vi "PC_SetCommandTo_PLC.vi"(0 "VISA resource name":refnum<visa-resource-name>, 1 "Mode":enum16{"RTU", "ASCII"}(ring), 2 "PLC Address":u8, 3 "Resistor":i32, 4 "Selection":T1(ring), 5 "error in (no error)":errorcluster) -> (6 "VISA resource name out":refnum<visa-resource-name>, 8 "error out":errorcluster)   [LabVIEW 2015]
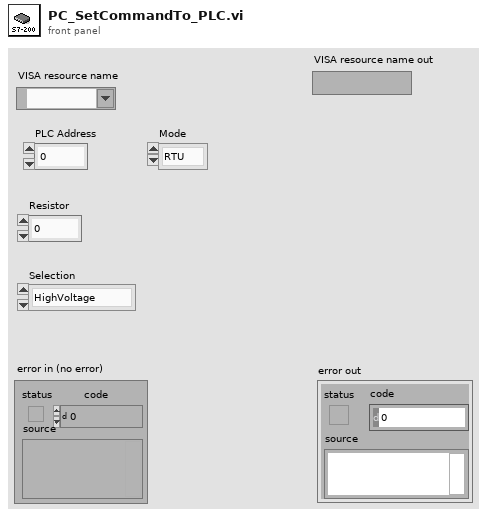
[diagram p1: front panel]
types:
  T1 = enum16{"HighVoltage", "LowVoltage", "Temperature", "AllOFF"}
  T2 = cluster{"Mode":enum16{"RTU", "ASCII"}, "Slave Address":u8}
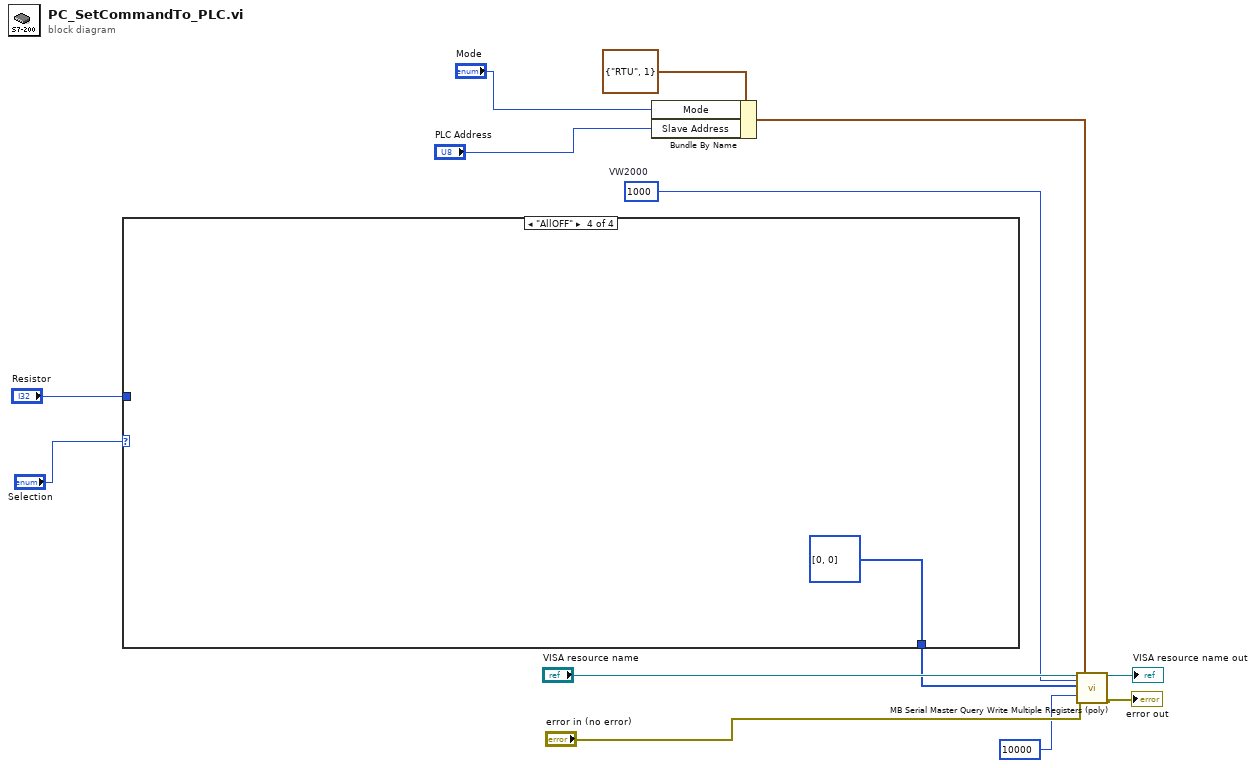
[diagram p0: block diagram]
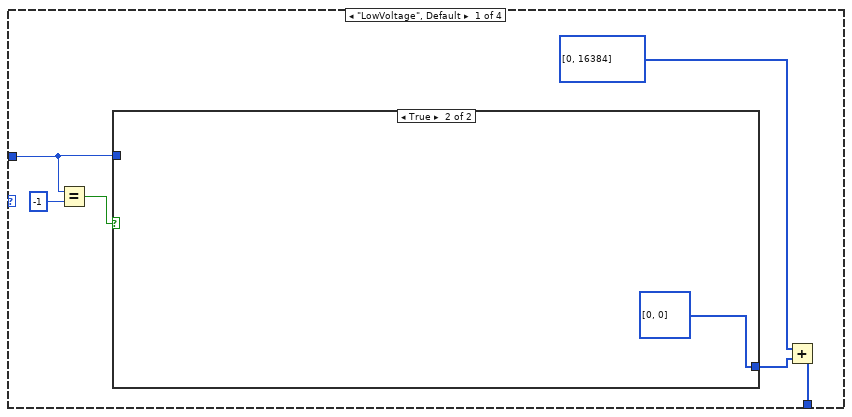
[diagram p2: hidden frame]
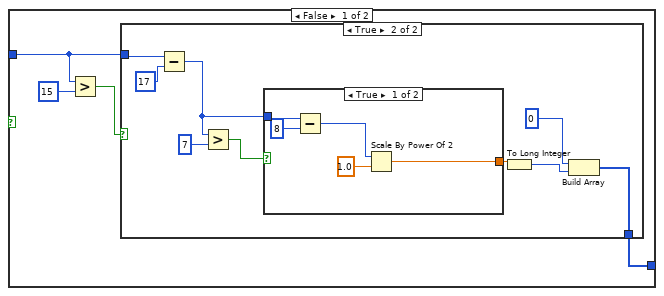
[diagram p3: hidden frame]
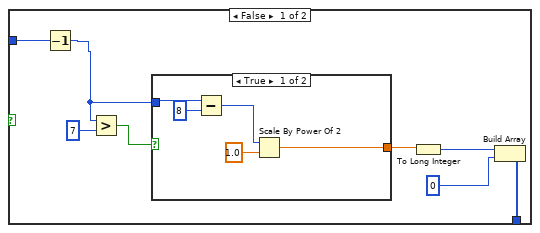
[diagram p4: hidden frame]
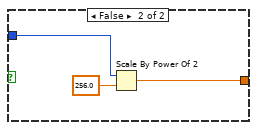
[diagram p5: hidden frame]
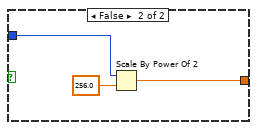
[diagram p6: hidden frame]
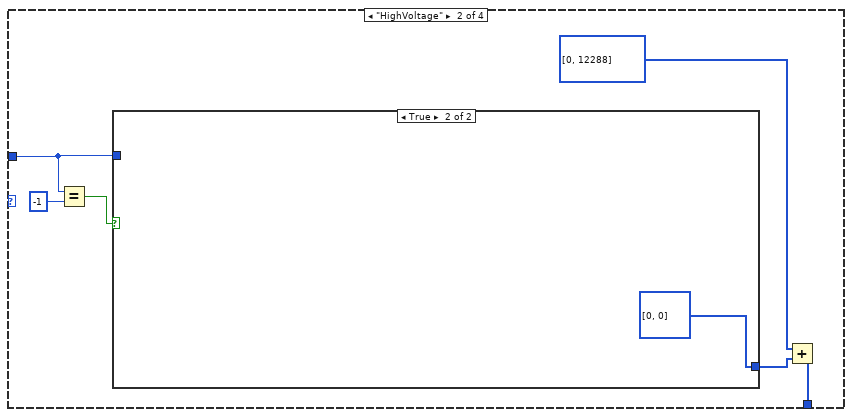
[diagram p7: hidden frame]
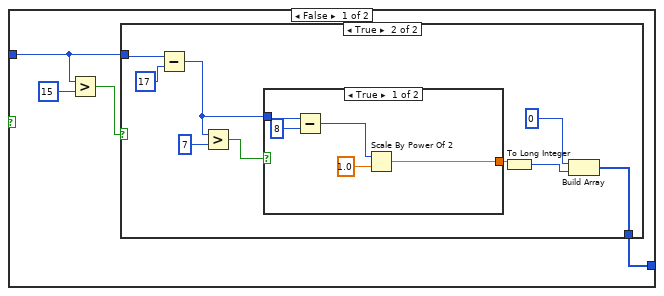
[diagram p8: hidden frame]
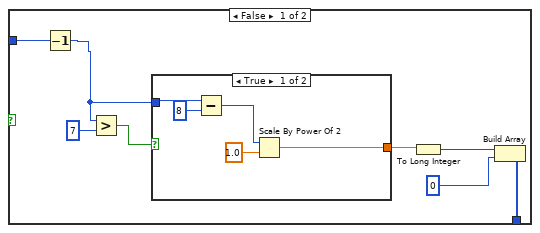
[diagram p9: hidden frame]
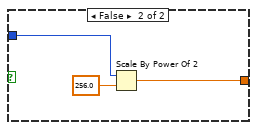
[diagram p10: hidden frame]
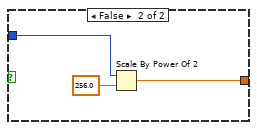
[diagram p11: hidden frame]
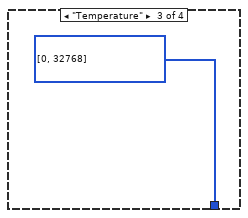
[diagram p12: hidden frame]
diagram:
  w4 = u16 1000  # VW2000
  n1 = case shown="\"AllOFF\"" "Selection" {
    tunnel: "Resistor" -> [w17 w61 _ _]
    tunnel: [w14 w58 i32[] [0, 32768] i32[] [0, 0]] -> w1
    frame "LowVoltage", Default {
      n2 = Equal?(x=w17, y=-1) -> (x = y?=w18:bool)
      n3 = case shown="True" w18 {
        tunnel: w17 -> [w21 _]
        tunnel: [w20 i32[] [0, 0]] -> w16
        frame False {
          n4 = Greater?(x=w21, y=15) -> (0:w22:bool)
          n5 = case shown="True" w22 {
            tunnel: w21 -> [w25 w42]
            tunnel: [w26 w45] -> w20
            frame False {
              n6 = Decrement(x=w25) -> (x-1=w24:i32)
              n7 = Greater?(x=w24, y=7) -> (0:w30:bool)
              n8 = case shown="True" w30 {
                tunnel: w24 -> [w34 w38]
                tunnel: [w35 w37] -> w29
                frame True {
                  n9 = Subtract(x=w34, y=8) -> (x-y=w32:i32)
                  n10 = Scale By Power Of 2(n=w32, x=1.0) -> (x*2^n=w35:dbl)
                }
                frame False {
                  n11 = Scale By Power Of 2(n=w38, x=256.0) -> (x*2^n=w37:dbl)
                }
              }
              n12 = To Long Integer(number=w29) -> (32bit integer=w28:i32)
              n13 = Build Array(w28, 0) -> (w26:i32[])
            }
            frame True {
              n14 = Subtract(x=w42, y=17) -> (x-y=w40:i32)
              n15 = Greater?(x=w40, y=7) -> (0:w47:bool)
              n16 = case shown="True" w47 {
                tunnel: w40 -> [w51 w55]
                tunnel: [w52 w54] -> w46
                frame True {
                  n17 = Subtract(x=w51, y=8) -> (x-y=w49:i32)
                  n18 = Scale By Power Of 2(n=w49, x=1.0) -> (x*2^n=w52:dbl)
                }
                frame False {
                  n19 = Scale By Power Of 2(n=w55, x=256.0) -> (x*2^n=w54:dbl)
                }
              }
              n20 = To Long Integer(number=w46) -> (32bit integer=w44:i32)
              n21 = Build Array(0, w44) -> (w45:i32[])
            }
          }
        }
        frame True {
        }
      }
      n22 = Add(x=i32[] [0, 16384], y=w16) -> (x+y=w14:i32[])
    }
    frame "HighVoltage" {
      n23 = Equal?(x=w61, y=-1) -> (x = y?=w62:bool)
      n24 = case shown="True" w62 {
        tunnel: w61 -> [w65 _]
        tunnel: [w64 i32[] [0, 0]] -> w60
        frame False {
          n25 = Greater?(x=w65, y=15) -> (0:w66:bool)
          n26 = case shown="True" w66 {
            tunnel: w65 -> [w69 w86]
            tunnel: [w70 w89] -> w64
            frame False {
              n27 = Decrement(x=w69) -> (x-1=w68:i32)
              n28 = Greater?(x=w68, y=7) -> (0:w74:bool)
              n29 = case shown="True" w74 {
                tunnel: w68 -> [w78 w82]
                tunnel: [w79 w81] -> w73
                frame True {
                  n30 = Subtract(x=w78, y=8) -> (x-y=w76:i32)
                  n31 = Scale By Power Of 2(n=w76, x=1.0) -> (x*2^n=w79:dbl)
                }
                frame False {
                  n32 = Scale By Power Of 2(n=w82, x=256.0) -> (x*2^n=w81:dbl)
                }
              }
              n33 = To Long Integer(number=w73) -> (32bit integer=w72:i32)
              n34 = Build Array(w72, 0) -> (w70:i32[])
            }
            frame True {
              n35 = Subtract(x=w86, y=17) -> (x-y=w84:i32)
              n36 = Greater?(x=w84, y=7) -> (0:w91:bool)
              n37 = case shown="True" w91 {
                tunnel: w84 -> [w95 w99]
                tunnel: [w96 w98] -> w90
                frame True {
                  n38 = Subtract(x=w95, y=8) -> (x-y=w93:i32)
                  n39 = Scale By Power Of 2(n=w93, x=1.0) -> (x*2^n=w96:dbl)
                }
                frame False {
                  n40 = Scale By Power Of 2(n=w99, x=256.0) -> (x*2^n=w98:dbl)
                }
              }
              n41 = To Long Integer(number=w90) -> (32bit integer=w88:i32)
              n42 = Build Array(0, w88) -> (w89:i32[])
            }
          }
        }
        frame True {
        }
      }
      n43 = Add(x=i32[] [0, 12288], y=w60) -> (x+y=w58:i32[])
    }
    frame "Temperature" {
    }
    frame "AllOFF" {
    }
  }
  n44 = Bundle By Name(cluster=T2 {"Mode"=enum."RTU", "Slave Address"=1} ("Serial Parameters"), "Mode"="Mode", "Slave Address"="PLC Address") -> (w7:T2)
  n45 = call "MB Serial Master Query Write Multiple Registers (poly).vi"("VISA resource name"="VISA resource name", "Starting Address"=w4, "Registers"=w1, "Timeout"=u32 10000, "error in"="error in (no error)", "Serial Parameters"=w7) -> ("VISA resource name out"=→"VISA resource name out":refnum<visa-resource-name>, "error out"=→"error out":errorcluster)  [unwired: 11 in, 1 out]
